vi "Store Static VI References for Subpanel.vi"(8 "error in (no error)":errorcluster, 11 "Client Config in":refnum<class "Client Config.lvclass">) -> (0 "error out":errorcluster, 3 "Client Config out":refnum<class "Client Config.lvclass">)   [LabVIEW 2017, in "Client Controller.lvlib" / "Client Config.lvclass"]
uses:
  Client Config.lvclass
  \\Mac\Home/Documents/Extensible-Config-Dialog/Configuration.lvclass
  <userlib>/Common Components/Msmt Configuration/Controller Configuration.lvclass
  <userlib>/Configuration Dialog Actor/Configuration.lvclass
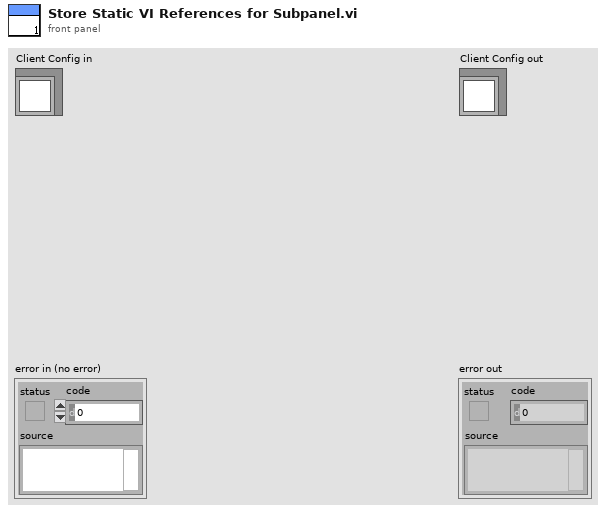
[diagram p1: front panel]
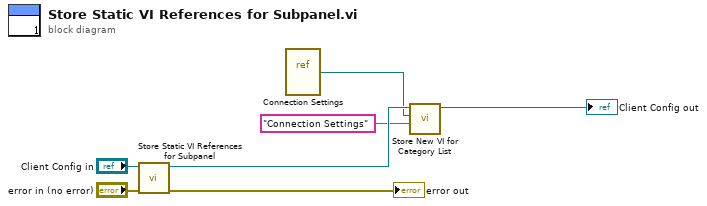
[diagram p0: block diagram]
diagram:
  n1 = call-parent "Store Static VI References for Subpanel.vi"("error in (no error)"="error in (no error)", "Controller Configuration in"="Client Config in") -> ("error out"=→"error out":errorcluster, "Controller Configuration out"=w4:refnum<class "Client Config.lvclass">)  [unwired: 8 in]
  n2 = vi-ref "Connection Settings.vi"() -> (w1:refnum<vi>)
  n3 = call <userlib>:"Store New VI for Category List.vi"("String"="Connection Settings", "VI Refnum"=w1, "Configuration in"=w4) -> ("Configuration out"=→"Client Config out":refnum<class "Client Config.lvclass">)  [unwired: 7 in, 1 out]
